vi "Code_to_run.vi"(1 "Open Front Panel":bool, 2 "Raw data option":enum16{"Save raw data", "Raw data not saved"}(ring), 3 "Acquisition Interlock":bool, 5 "setup":T3, 7 "Remote control":bool, 9 "File":T1, 11 "Results Filename":path, 12 "Raw data file":path, 13 "Averaging time (min)":dbl=6.0 format="%.2f", 14 "Setup filename":string) -> (15 "Status":T2)   [LabVIEW 2010]
uses:
  Controls/Setup.ctl
  Multi_Run_Status.ctl
  Controls/Save_Data.ctl
  Controls/Post_Process.ctl
  Globals/Trav_pos_global.vi
  Globals/Dynamic_call_global.ph.vi
  Globals/Meas_global.vi
  Globals/Constants_global.vi
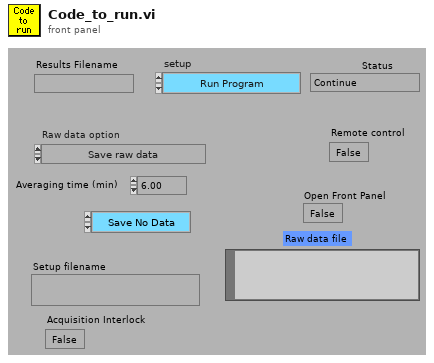
[diagram p1: front panel]
types:
  T1 = typedef "Save_Data.ctl" = enum16{"Save No Data", "Save Data"}
  T2 = typedef "Multi_Run_Status.ctl" = enum16{"Continue", "Jump to Next Point", "Jump to Next Row", "Jump To Fall Back", "Terminate Run"}
  T3 = typedef "Setup.ctl" = enum16{"Run Program", "Show Setup", "Save Current Setup", "Setup Front Panel"}
  T4 = typedef "Traverse_cluster.ctl" = cluster{"Start X":dbl, "Start Y":dbl, "Start Z":dbl, "End X":dbl, "End Y":dbl, "End Z":dbl, "No. of pts.":i32, "Spacing":T5, "Filename":path, "Tunnel Speed":dbl, "Averaging time (min)":dbl, "Extra Commands":string, "Specific Arguments":string, "Emission Rate (l/min)":dbl, "Trace Gas Concentration (%)":dbl, "Density Ratio":string, "Comments":string, "Row No":i32, "Row Type Selector":T6, "Completion time":string, "Row Duration (mins)":dbl, "No. of Valid pts.":i32, "Meas Setup File":string}
  T5 = typedef "Spacing.ctl" = enum16{"Linear", "Log", "Gauss", "Specified", "N/A"}
  T6 = typedef "Multi_run_mode.ctl" = enum16{"Move Traverse Only", "Set Tunnel Speed Only", "Set Source Only", "Set Measurement Conditions", "Single Measurement", "Vertical Profile", "Lateral Profile", "Longitudinal Profile", "Explore Volume", "Multi-Axis Profile", "Auto Calibrate", "Meas Fast FID Bkgnd", "Check Beam Power", "Scanning Valve Measurement", "Run VI Named:", "Set ADAM Ch", "Wait (minutes)", "Send Message", "Synchronize With:", "Fall Back to this Row", "Turn Off Row Repeating", "Blank Row"}
  T7 = typedef "Post_Process.ctl" = enum16{"Take New Data", "Post Process Raw Data File"}
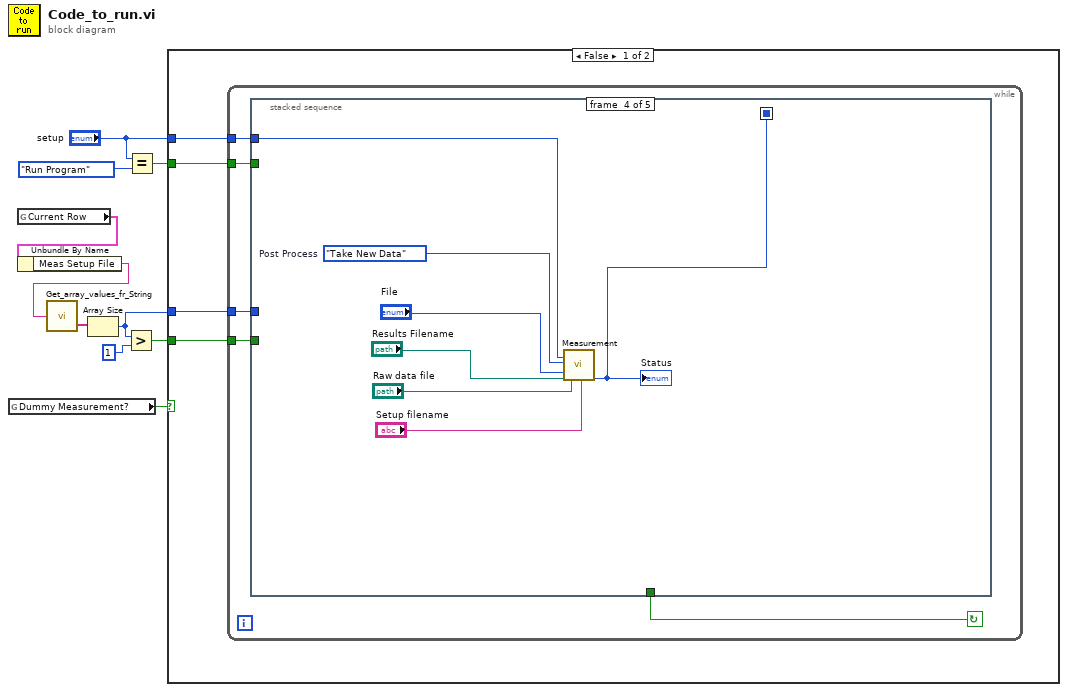
[diagram p0: block diagram]
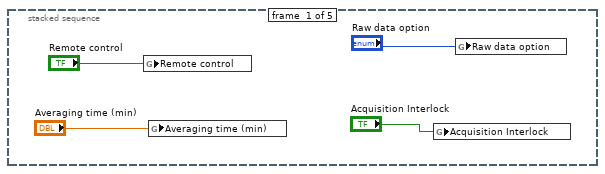
[diagram p2: hidden frame]
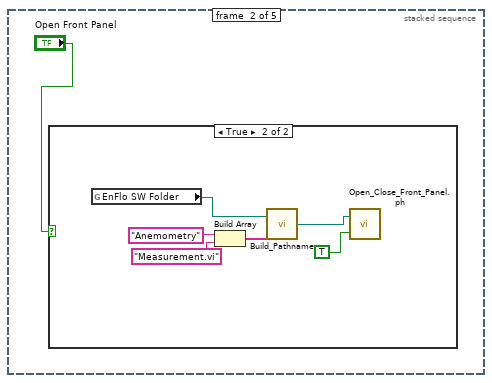
[diagram p3: hidden frame]
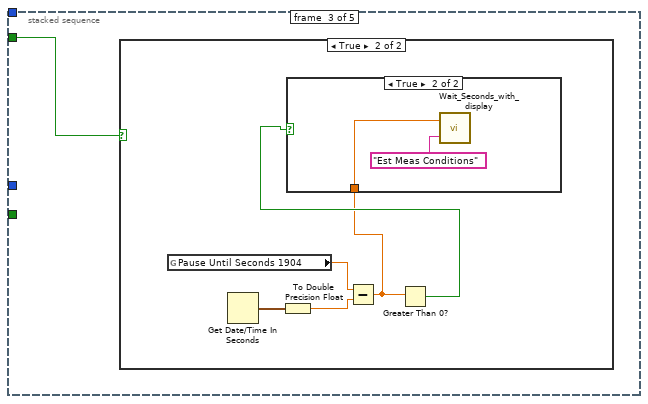
[diagram p5: hidden frame]
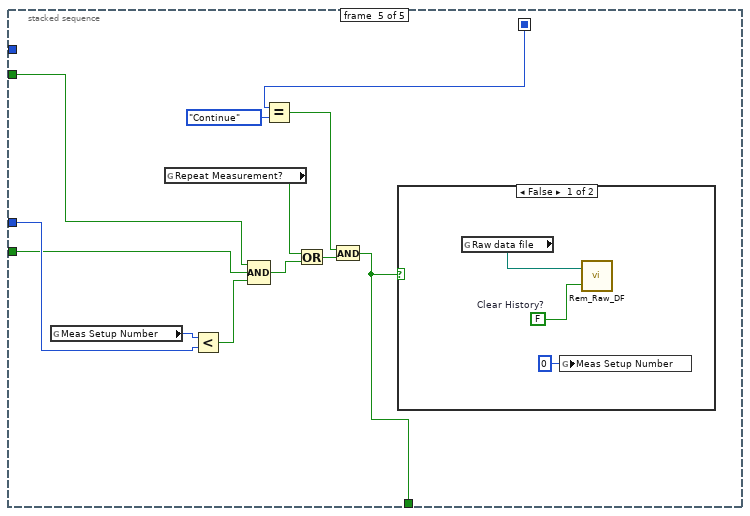
[diagram p8: hidden frame]
diagram:
  n1 = global read "Trav_pos_global.vi" "Dummy Measurement?"() -> (w10:bool)
  n2 = global read "Trav_pos_global.vi" "Current Row"() -> (w9:T4)
  n3 = Unbundle By Name(w9) -> ("Meas Setup File"=w8:string)
  n4 = call "Get_array_values_fr_String.vi"("String Value"=w8) -> ("String array"=w7:string[])  [unwired: 1 out]
  n5 = Array Size(array=w7) -> (size(s)=w5:i32)
  n6 = Greater?(x=w5, y=1) -> (0:w4:bool)
  n7 = Equal?(x="setup", y=Setup."Run Program" ("setup")) -> (x = y?=w1:bool)
  n8 = case shown="False" w10 {
    tunnel: w5 -> [w14 _]
    tunnel: w4 -> [w13 _]
    tunnel: "setup" -> [w12 _]
    tunnel: w1 -> [w11 _]
    frame False {
      n9 = while {
        tunnel: w14 -> [w18]
        tunnel: w13 -> [w17]
        tunnel: w12 -> [w16]
        tunnel: w11 -> [w15]
        stop <- w19 continue-if-true
        n10 = stacked-sequence {
          seq-local: [_ _ _ w40 _] -> [_ _ _ _ w56]
          tunnel: [_ _ _ _ w47] -> w19
          tunnel: w18 -> [_ _ _ _ w54]
          tunnel: w17 -> [_ _ _ _ w52]
          tunnel: w16 -> [_ _ _ w39 _]
          tunnel: w15 -> [_ _ w31 _ w46]
          frame #0 {
            n11 = global write "Meas_global.vi" "Remote control"("Remote control") -> ()
            n12 = global write "Meas_global.vi" "Averaging time (min)"("Averaging time (min)") -> ()
            n13 = global write "Dynamic_call_global.ph.vi" "Acquisition Interlock"("Acquisition Interlock") -> ()
            n14 = global write "Meas_global.vi" "Raw data option"("Raw data option") -> ()
          }
          frame #1 {
            n15 = case shown="True" "Open Front Panel" {
              frame False {
              }
              frame True {
                n16 = global read "Constants_global.vi" "EnFlo SW Folder"() -> (w27:path)
                n17 = Build Array("Anemometry", "Measurement.vi") -> (w28:string[])
                n18 = call "Build_Pathname.vi"("Output Array"=w28, "Pathname"=w27) -> ("Appended path"=w26:path)
                n19 = call "Open_Close_Front_Panel.ph.vi"("Front Panel Window:Open"=TRUE, "VI path"=w26) -> ()  [unwired: 2 out]
              }
            }
          }
          frame #2 {
            n20 = case shown="True" w31 {
              frame False {
              }
              frame True {
                n21 = global read "Trav_pos_global.vi" "Pause Until Seconds 1904"() -> (w36:dbl)
                n22 = Get Date/Time In Seconds() -> (seconds since 1Jan1904=w35:timestamp)
                n23 = To Double Precision Float(number=w35) -> (double precision float=w34:dbl)
                n24 = Subtract(x=w36, y=w34) -> (x-y=w32:dbl)
                n25 = Greater Than 0?(x=w32) -> (x > 0?=w33:bool)
                n26 = case shown="True" w33 {
                  tunnel: w32 -> [_ w37]
                  frame False {
                  }
                  frame True {
                    n27 = call "Wait_Seconds_with_display.vi"("Message"="Est Meas Conditions", "Seconds to wait"=w37) -> ()  [unwired: 2 out]
                  }
                }
              }
            }
          }
          frame #3 {
            w41 = Post_Process."Take New Data"  # Post Process
            n28 = call "Measurement.vi"("setup"=w39, "Post Process"=w41, "File"="File", "Results file"="Results Filename", "Raw data file"="Raw data file", "Setup filename"="Setup filename") -> ("Status Out"=w40:T2)  [unwired: 1 in, 12 out]
            "Status" <- w40
          }
          frame #4 {
            n29 = global read "Trav_pos_global.vi" "Meas Setup Number"() -> (w55:i32)
            n30 = global read "Meas_global.vi" "Repeat Measurement?"() -> (w50:bool)
            n31 = Less?(x=w55, y=w54) -> (x < y?=w53:bool)
            n32 = Compound Arithmetic op=AND(w46, w52, w53) -> (w51:bool)
            n33 = Equal?(x=w56, y=Multi_Run_Status."Continue" ("Status Out")) -> (x = y?=w48:bool)
            n34 = Or(x=w50, y=w51) -> (x .or. y?=w49:bool)
            n35 = And(x=w48, y=w49) -> (x .and. y?=w47:bool)
            n36 = case shown="False" w47 {
              frame False {
                w59 = FALSE  # Clear History?
                n37 = global read "Meas_global.vi" "Raw data file"() -> (w60:path)
                n38 = global write "Trav_pos_global.vi" "Meas Setup Number"(0 ("Meas Setup Number")) -> ()
                n39 = call "Rem_Raw_DF.vi"("Clear History?"=w59, "Filename to Remember"=w60) -> ()  [unwired: 1 out]
              }
              frame True {
              }
            }
          }
        }
      }
    }
    frame True {
    }
  }
